vi "Acknowledge Post Process.vi"(8 "error in (no error)":errorcluster, 10 "Ack Result":refnum<class "Acquired Result.lvclass">, 11 "Monitor-Pulse in":refnum<class "Monitor-Pulse.lvclass">) -> (0 "error out":errorcluster, 3 "Monitor-Pulse out":refnum<class "Monitor-Pulse.lvclass">)   [LabVIEW 2015, in "Monitor-Pulse.lvclass"]
uses:
  Monitor-Pulse.lvclass
  Measure_core/Results/Acquired Result/Acquired Result.lvclass
  Measure_core/Process Object Messages/Process Result Msg/Process Result Msg.lvclass/Process Result Msg.ctl
  <vilib>/ActorFramework/Message Enqueuer/Message Enqueuer.lvclass/Message Enqueuer.ctl
  <vilib>/ActorFramework/Message Enqueuer/Enqueue.vi
  <vilib>/ActorFramework/Message Priority Queue/Priority Enqueue.vi
  Measure_core/Process Object Messages/Process Result Msg/Process Result Msg.lvclass
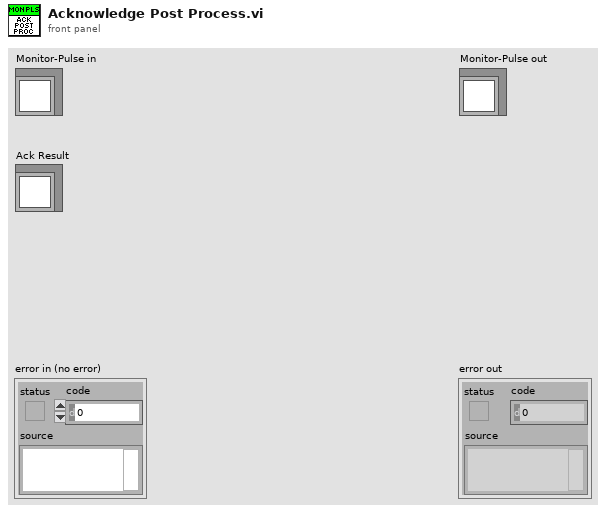
[diagram p1: front panel]
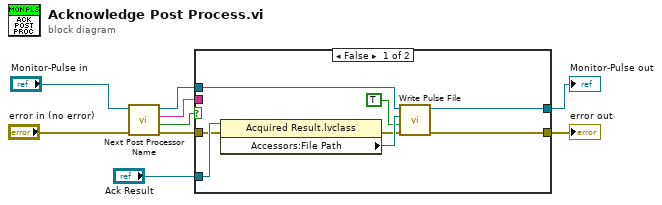
[diagram p0: block diagram]
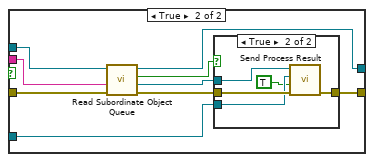
[diagram p2: hidden frame]
diagram:
  n1 = call-dynamic "Next Post Processor Name.vi"("error in (no error)"="error in (no error)", "Monitor-Pulse in"="Monitor-Pulse in") -> ("error out"=w4:errorcluster, "Valid name"=w2:bool, "Post processor name"=w6:string, "Monitor-Pulse out"=w7:refnum<class "Monitor-Pulse.lvclass">)  [unwired: 6 in]
  n2 = case shown="False" w2 {
    tunnel: w7 -> [w17 w26]
    tunnel: w6 -> [_ w25]
    tunnel: [w16 w21] -> w5
    tunnel: w4 -> [w11 w20]
    tunnel: [w15 w19] -> w3
    tunnel: "Ack Result" -> [w14 w18]
    frame False {
      n3 = property class="Acquired Result.lvclass"(reference=w14, error in=w11) -> (error out=w10:errorcluster, "Accessors:File Path"=w13:path)  [unwired: 1 out]
      n4 = call-dynamic "Write Pulse File.vi"("error in (no error)"=w10, "Open plot after pulse"=TRUE, "Pulse File"=w13, "Monitor-Pulse in"=w17) -> ("error out"=w15:errorcluster, "Monitor-Pulse out"=w16:refnum<class "Monitor-Pulse.lvclass">)  [unwired: 6 in]
    }
    frame True {
      n5 = call-dynamic "Read Subordinate Object Queue.vi"("error in (no error)"=w20, "Name"=w25, "Measure Object in"=w26) -> ("error out"=w23:errorcluster, "Object Enqueuer"=w22:refnum<class "Message Enqueuer.lvclass">, "Found?"=w24:bool, "Measure Object out"=w21:refnum<class "Monitor-Pulse.lvclass">)  [unwired: 5 in]
      n6 = case shown="True" w24 {
        tunnel: w22 -> [_ w32]
        tunnel: w23 -> [w27 w31]
        tunnel: [w27 w30] -> w19
        tunnel: w18 -> [_ w29]
        frame False {
        }
        frame True {
          n7 = call "Send Process Result.vi"("error in (no error)"=w31, "Acknowledge"=TRUE, "Result in"=w29, "Message Enqueuer"=w32) -> ("error out"=w30:errorcluster)  [unwired: 6 in, 1 out]
        }
      }
    }
  }
  "error out" <- w3
  "Monitor-Pulse out" <- w5
